vi "Keithley 6514 Buffer Math Config.vi"(0 "Resource In":refnum<visa-resource-name>, 1 "Check For SCPI Errors? (T)":bool=TRUE, 7 "calculation (mean:0)":u16(ring) items=["mean", "standard deviation", "maximum", "mimimum", "peak-to-peak"], 11 "error in (no error)":T1) -> (4 "Resource Out (dupl)":refnum<visa-resource-name>, 15 "error out":T1)   [LabVIEW 2014, in "KE6514Driver.lvlib"]
doc: "This VI is used to configure the settings for buffer math calculation 3. This involves operations on readings stored in the buffer.\n\nTo read the results of the calculation, use the Math Read VI."
uses:
  KE6514Driver.lvlib
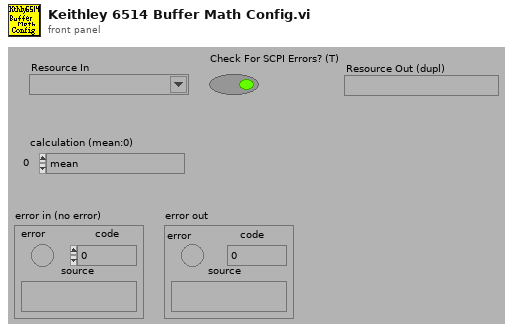
[diagram p1: front panel]
types:
  T1 = cluster{"error":bool, "code":i32, "source":string}
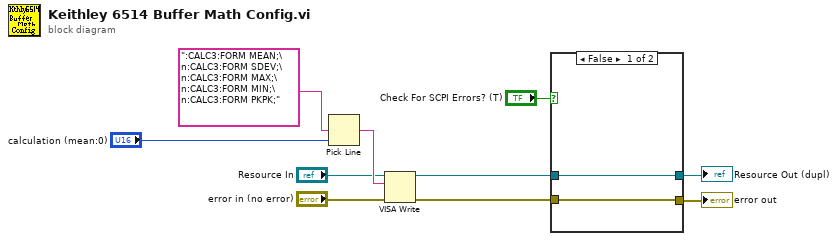
[diagram p0: block diagram]
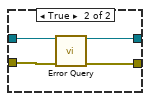
[diagram p2: hidden frame]
diagram:
  n1 = Pick Line(multi-line string=":CALC3:FORM MEAN;\n:CALC3:FORM SDEV;\n:CALC3:FORM MAX;\n:CALC3:FORM MIN;\n:CALC3:FORM PKPK;", line index="calculation (mean:0)") -> (output string=w8:string)  [unwired: 1 in]
  n2 = VISA Write(VISA resource name="Resource In", write buffer=w8, error in (no error)="error in (no error)") -> (VISA resource name out=w4:refnum<visa-resource-name>, error out=w3:errorcluster)  [unwired: 1 out]
  n3 = case shown="False" "Check For SCPI Errors? (T)" {
    tunnel: w4 -> [w12 w16]
    tunnel: w3 -> [w11 w15]
    tunnel: [w12 w14] -> w2
    tunnel: [w11 w13] -> w1
    frame False {
    }
    frame True {
      n4 = call "Error Query.vi"("VISA Resource In"=w16, "error in (no error)"=w15) -> ("VISA Resource Out (dupl)"=w14:refnum<visa-resource-name>, "error out"=w13:errorcluster)  [unwired: 10 in, 2 out]
    }
  }
  "error out" <- w1
  "Resource Out (dupl)" <- w2
